vi "Labview_Fire_Alarm_Adruino.vi"() -> ()   [LabVIEW 2021]
uses:
  <vilib>/MakerHub/LINX/Public/Peripherals/Analog/Analog Read 1 Chan.vi
  <vilib>/MakerHub/LINX/Public/Peripherals/Digital/Digital Write 1 Chan.vi
  <vilib>/MakerHub/LINX/Public/Peripherals/Digital/Digital Read 1 Chan.vi
  <vilib>/MakerHub/LINX/Public/Peripherals/Analog/Analog Read N Chans.vi
  <vilib>/MakerHub/LINX/Public/Peripherals/Digital/Digital Write N Chans.vi
  <vilib>/MakerHub/LINX/Public/Peripherals/Digital/Digital Read N Chans.vi
  <vilib>/MakerHub/LINX/Private/Local IO/LinxAnalogRead.vi
  <vilib>/MakerHub/LINX/Public/Utilities/Check Channel.vi
  <vilib>/MakerHub/LINX/Private/Local IO/LinxDigitalWrite.vi
  <vilib>/MakerHub/LINX/Private/Local IO/LinxDigitalRead.vi
  <vilib>/MakerHub/LINX/Public/Utilities/Open Serial.vi
  <vilib>/MakerHub/LINX/Private/Utilties/Generate Error.vi
  <vilib>/MakerHub/LINX/Public/Sensors/Motion/Servo/Servo Open One Channel.vi
  <vilib>/MakerHub/LINX/Public/Sensors/Motion/Servo/Servo Set Pulse Width One Channel.vi
  <vilib>/MakerHub/LINX/Public/Sensors/Motion/Servo/Servo Close One Channel.vi
  <vilib>/MakerHub/LINX/LMH-LINX.lvlib
  <vilib>/MakerHub/LINX/Public/Sensors/Motion/Servo/Servo.lvlib
panel:
  in  "stop 2":bool
  out "DOOR":bool
  in  "stop 3":bool
  out "Qua nhiet do 2":bool
  out "Nhiet do 3":dbl(graph)
  out "Nhiet do 2":dbl(slide) scale=0.0..100.0
  in  "Nhiet do dat 2":dbl
  out "Nhiet do phong  2":dbl
  out "ppm":dbl
  out "Rs":dbl
  out "Thoi gian thuc":timestamp
  in  "Serial Port":refnum<visa-resource-name>="N/A"
  out "Warning gas (uzz)":bool
  out "Quat":bool
  in  "Nguong canh bao":dbl
  out "Smoke Output":dbl(knob) scale=0.0..1025.0
  in  "stop":bool
  # "CANH BAO KHI GAS"
  # "CANH BAO NHIET DO"
  # "CUA TU DONG"
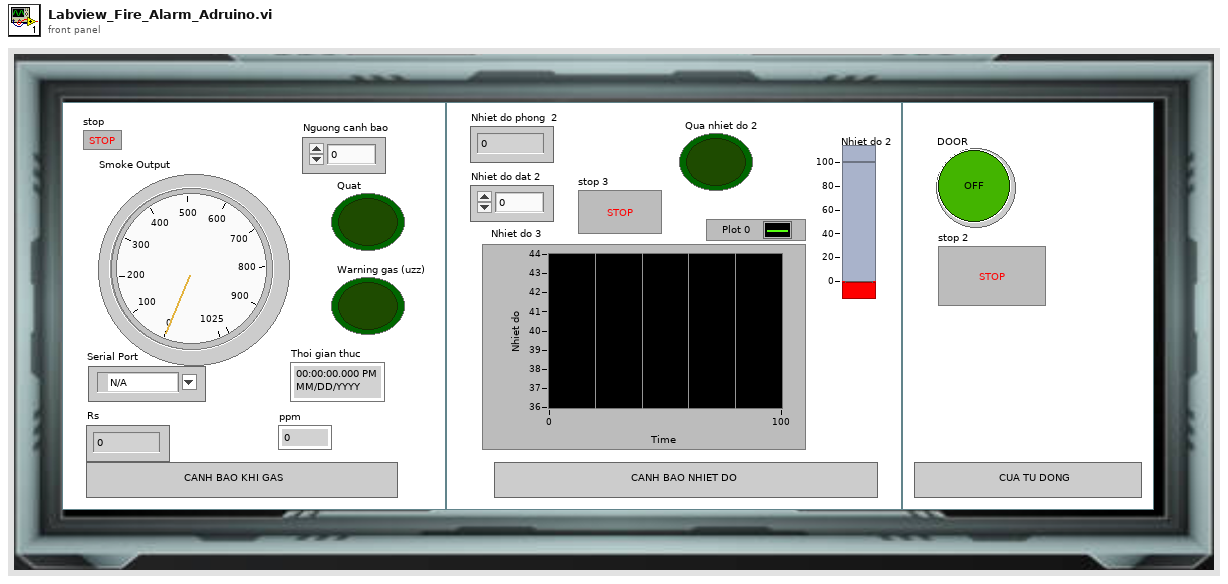
[diagram p1: front panel]
types:
  T1 = typedef "LMH-LINX.lvlib/LINX Ref.ctl" = cluster{"IO":T2, "Interface":T3, "LINX Device Config":T4}
  T2 = typedef "LMH-LINX.lvlib/Platform.ctl" = enum16{"Remote", "Local"}
  T3 = typedef "LMH-LINX.lvlib/Interface.ctl" = enum16{"Serial", "TCP"}
  T4 = typedef "LMH-LINX.lvlib/Device.lvlib/LINX Device Config.ctl" = cluster{"Interface":T3, "COM Port":refnum<visa-resource-name>, "TCP Configuration":T5, "Device Family":u8, "Device ID":u8, "Device Name":string, "TCP Ref":refnum<k5>, "Channels":T6}
  T5 = typedef "LMH-LINX.lvlib/Device.lvlib/TCP Config.ctl" = cluster{"IP Address":string, "Port":u16}
  T6 = typedef "LMH-LINX.lvlib/Channels.ctl" = cluster{"DI":u8[], "DO":u8[], "AI":u8[], "AO":u8[], "PWM":u8[], "QE":u8[], "UART":u8[], "I2C 2":u8[], "SPI":u8[], "CAN":u8[], "Servo":u8[], "AI Ref (V)":dbl, "AI Resolution (Bits)":u8, "AO Ref (V)":dbl, "AO Resolution (Bits)":u8}
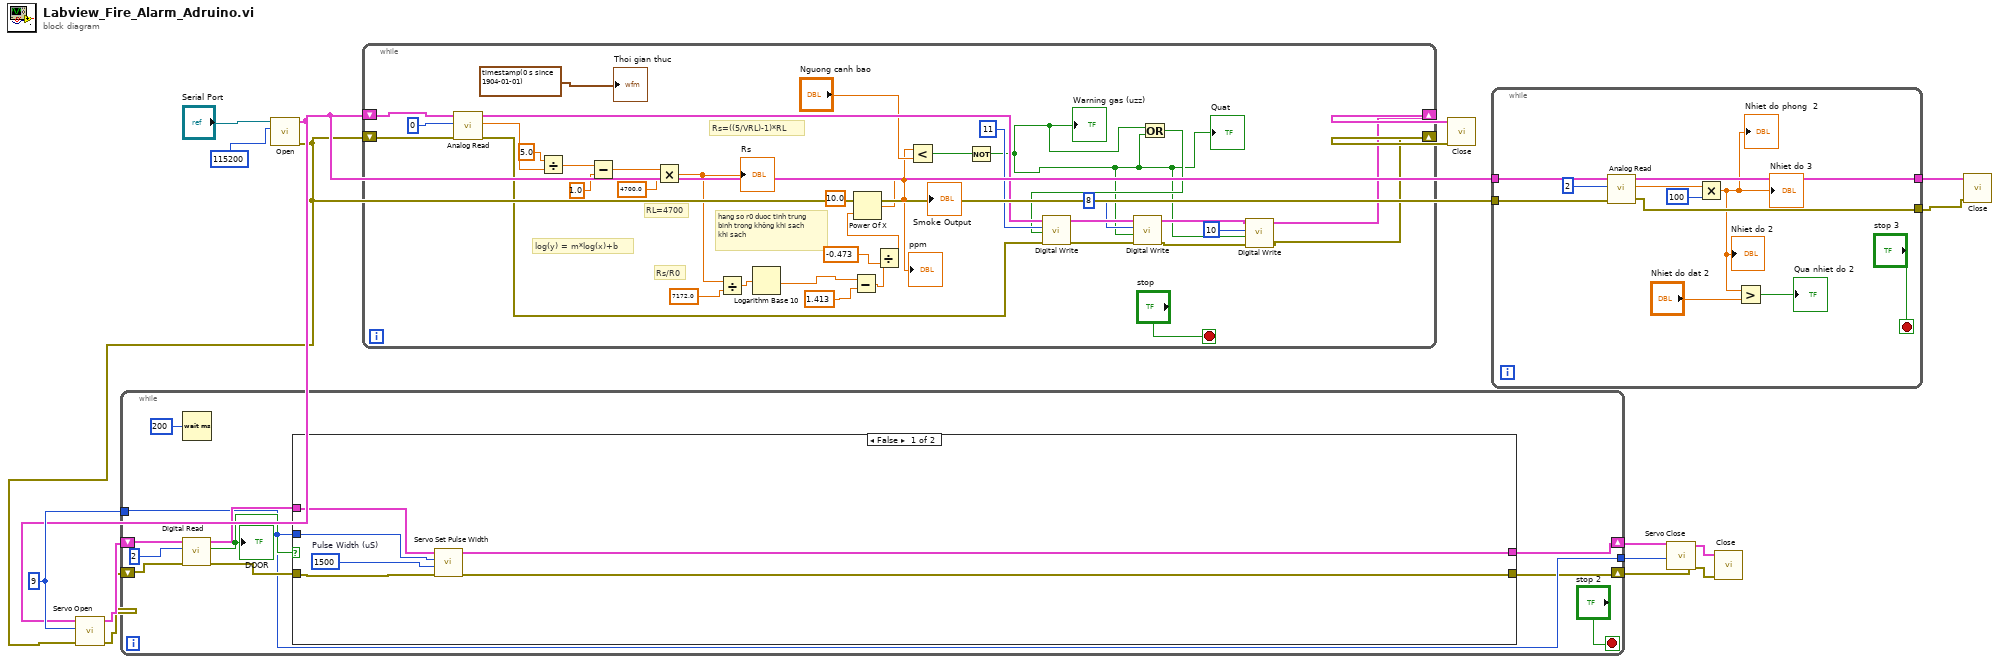
[diagram p0: block diagram]
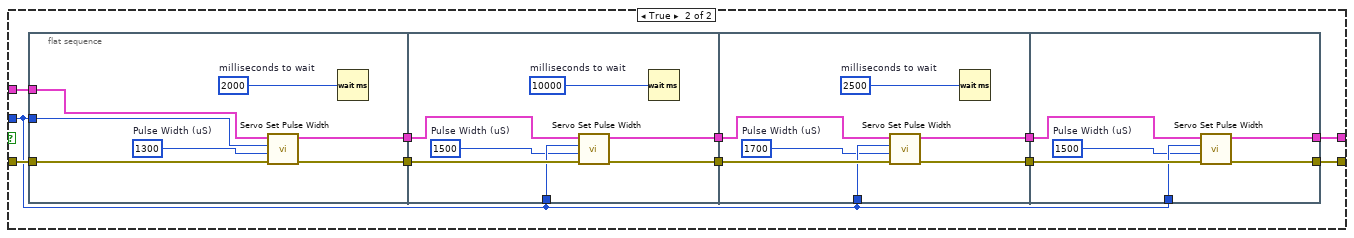
[diagram p2: hidden frame]
diagram:
  w6 = u8 9 ("Servo Channel")
  n1 = call-poly <vilib>:"Open.vi"("Baud Rate Override"=u32 115200, "Serial Port"="Serial Port") -> ("Error Out"=w1:errorcluster, "LINX Resource"=w2:T1)  [unwired: 7 in, 1 out]
  n2 = call-poly <vilib>:"Servo Open.vi"("Error In"=w1, "Servo Channel"=w6, "LINX Resource"=w2) -> ("Error Out"=w3:errorcluster, "LINX Resource"=w4:T1)  [unwired: 7 in]
  n3 = while {
    shift-right: [w18] -> w10
    shift-left: w4 -> [w19]
    shift-right: [w17] -> w9
    shift-left: w3 -> [w26]
    tunnel: w6 -> [w21]
    tunnel: [w21] -> w5
    stop <- "stop 2" stop-if-true
    n4 = call-poly <vilib>:"Digital Read.vi"("Error In"=w26, "DI Channel"=u8 2, "LINX Resource"=w19) -> ("Error Out"=w22:errorcluster, "DI Value"=w24:bool, "LINX Resource"=w23:T1)  [unwired: 6 in]
    "DOOR" <- w24
    n5 = Wait (ms)(milliseconds to wait=u32 200) -> ()  [unwired: 1 out]
    n6 = case shown="False" w24 {
      tunnel: w23 -> [w32 w44]
      tunnel: w22 -> [w33 w43]
      tunnel: w21 -> [w31 w36]
      tunnel: [w29 w35] -> w17
      tunnel: [w28 w34] -> w18
      frame False {
        w30 = u16 1500  # Pulse Width (uS)
        n7 = call-poly <vilib>:"Servo Set Pulse Width.vi"("Error In"=w33, "Pulse Width (uS)"=w30, "Servo Channel"=w31, "LINX Resource"=w32) -> ("Error Out"=w29:errorcluster, "LINX Resource"=w28:T1)  [unwired: 6 in]
      }
      frame True {
        n8 = flat-sequence {
          tunnel: w44 -> [w51]
          tunnel: w43 -> [w50]
          tunnel: [w49] -> w42
          tunnel: [w48] -> w41
          tunnel: w36 -> [w46]
          tunnel: w42 -> [w58]
          tunnel: w41 -> [w57]
          tunnel: [w56] -> w40
          tunnel: [w55] -> w39
          tunnel: w36 -> [w54]
          tunnel: w40 -> [w65]
          tunnel: w39 -> [w64]
          tunnel: [w63] -> w38
          tunnel: [w62] -> w37
          tunnel: w36 -> [w61]
          tunnel: w38 -> [w71]
          tunnel: w37 -> [w70]
          tunnel: [w69] -> w34
          tunnel: [w68] -> w35
          tunnel: w36 -> [w67]
          frame #0 {
            w45 = u16 1300  # Pulse Width (uS)
            w47 = u32 2000  # milliseconds to wait
            n9 = call-poly <vilib>:"Servo Set Pulse Width.vi"("Error In"=w50, "Pulse Width (uS)"=w45, "Servo Channel"=w46, "LINX Resource"=w51) -> ("Error Out"=w49:errorcluster, "LINX Resource"=w48:T1)  [unwired: 6 in]
            n10 = Wait (ms)(milliseconds to wait=w47) -> ()  [unwired: 1 out]
          }
          frame #1 {
            w52 = u32 10000  # milliseconds to wait
            w53 = u16 1500  # Pulse Width (uS)
            n11 = call-poly <vilib>:"Servo Set Pulse Width.vi"("Error In"=w58, "Pulse Width (uS)"=w53, "Servo Channel"=w54, "LINX Resource"=w57) -> ("Error Out"=w55:errorcluster, "LINX Resource"=w56:T1)  [unwired: 6 in]
            n12 = Wait (ms)(milliseconds to wait=w52) -> ()  [unwired: 1 out]
          }
          frame #2 {
            w59 = u32 2500  # milliseconds to wait
            w60 = u16 1700  # Pulse Width (uS)
            n13 = call-poly <vilib>:"Servo Set Pulse Width.vi"("Error In"=w64, "Pulse Width (uS)"=w60, "Servo Channel"=w61, "LINX Resource"=w65) -> ("Error Out"=w62:errorcluster, "LINX Resource"=w63:T1)  [unwired: 6 in]
            n14 = Wait (ms)(milliseconds to wait=w59) -> ()  [unwired: 1 out]
          }
          frame #3 {
            w66 = u16 1500  # Pulse Width (uS)
            n15 = call-poly <vilib>:"Servo Set Pulse Width.vi"("Error In"=w70, "Pulse Width (uS)"=w66, "Servo Channel"=w67, "LINX Resource"=w71) -> ("Error Out"=w68:errorcluster, "LINX Resource"=w69:T1)  [unwired: 6 in]
          }
        }
      }
    }
  }
  n16 = while {
    shift-right: [w75] -> w14
    shift-left: w2 -> [w88]
    shift-right: [w74] -> w13
    shift-left: w1 -> [w87]
    stop <- "stop" stop-if-true
    # "log(y) = m*log(x)+b"
    # "Rs/R0"
    # "hang so r0 duoc tinh trung binh trong không khi sach\nkhi sach"
    # "RL=4700"
    # "Rs=((5/VRL)-1)*RL"
    n17 = call-poly <vilib>:"Analog Read.vi"("Error In"=w87, "Analog Channel"=u8 0, "LINX Resource"=w88) -> ("Error Out"=w107:errorcluster, "Voltage"=w95:dbl, "LINX Resource"=w106:T1)  [unwired: 5 in, 1 out]
    n18 = Divide(x=5.0, y=w95) -> (x/y=w94:dbl)
    n19 = Subtract(x=w94, y=1.0) -> (x-y=w92:dbl)
    n20 = Multiply(x=w92, y=4700.0) -> (x*y=w90:dbl)
    "Rs" <- w90
    n21 = Divide(x=w90, y=7172.0) -> (x/y=w86:dbl)
    n22 = Logarithm Base 10(1:w86) -> (0:w85:dbl)
    n23 = Subtract(x=w85, y=1.413) -> (x-y=w82:dbl)
    n24 = Divide(x=w82, y=-0.473 ("x")) -> (x/y=w80:dbl)
    n25 = Power Of X(1:w80, 2:10.0 ("y")) -> (0:w79:dbl)
    "Smoke Output" <- w79
    "ppm" <- w79
    n26 = Less?(x=w79, y="Nguong canh bao") -> (x < y?=w101:bool)
    n27 = Not(x=w101) -> (.not. x?=w72:bool)
    "Quat" <- w72
    "Warning gas (uzz)" <- w72
    n28 = Or(x=w72, y=w72) -> (x .or. y?=w73:bool)
    n29 = call-poly <vilib>:"Digital Write.vi"("Error In"=w107, "Output Value"=w73, "DO Channel"=u8 11, "LINX Resource"=w106) -> ("Error Out"=w99:errorcluster, "LINX Resource"=w100:T1)  [unwired: 6 in]
    n30 = call-poly <vilib>:"Digital Write.vi"("Error In"=w99, "Output Value"=w72, "DO Channel"=u8 8, "LINX Resource"=w100) -> ("Error Out"=w76:errorcluster, "LINX Resource"=w77:T1)  [unwired: 6 in]
    n31 = call-poly <vilib>:"Digital Write.vi"("Error In"=w76, "Output Value"=w72, "DO Channel"=u8 10, "LINX Resource"=w77) -> ("Error Out"=w74:errorcluster, "LINX Resource"=w75:T1)  [unwired: 6 in]
    "Thoi gian thuc" <- timestamp(0 s since 1904-01-01)
  }
  n32 = call <vilib>:"Close.vi"("Error In"=w13, "LINX Resource"=w14) -> ()  [unwired: 9 in, 1 out]
  n33 = while {
    tunnel: w2 -> [w114]
    tunnel: w1 -> [w113]
    tunnel: [w112] -> w12
    tunnel: [w111] -> w11
    stop <- "stop 3" stop-if-true
    n34 = call-poly <vilib>:"Analog Read.vi"("Error In"=w113, "Analog Channel"=u8 2, "LINX Resource"=w114) -> ("Error Out"=w111:errorcluster, "Voltage"=w117:dbl, "LINX Resource"=w112:T1)  [unwired: 5 in, 1 out]
    n35 = Multiply(x=w117, y=100) -> (x*y=w109:dbl)
    "Nhiet do phong  2" <- w109
    "Nhiet do 2" <- w109
    "Nhiet do 3" <- w109
    n36 = Greater?(x=w109, y="Nhiet do dat 2") -> (0:→"Qua nhiet do 2":bool)
  }
  n37 = call-poly <vilib>:"Servo Close.vi"("Error In"=w9, "Servo Channel"=w5, "LINX Resource"=w10) -> ("Error Out"=w7:errorcluster, "LINX Resource"=w8:T1)  [unwired: 7 in]
  n38 = call <vilib>:"Close.vi"("Error In"=w7, "LINX Resource"=w8) -> ()  [unwired: 9 in, 1 out]
  n39 = call <vilib>:"Close.vi"("Error In"=w11, "LINX Resource"=w12) -> ()  [unwired: 9 in, 1 out]
